vi "Rational Resampling.vi"() -> ()   [LabVIEW 2020]
doc: "This example demonstrates how to use the Rational Resample VI to process a large data sequence consisting of smaller blocks."
uses:
  <vilib>/Utility/error.llb/DialogType.ctl
  <vilib>/Analysis/2dsp.llb/Rational Resample (single channel, DBL).vi
  <vilib>/Analysis/NI_AALPro.lvlib
  <vilib>/Analysis/NI_AALBase.lvlib
panel:
  out "error message":string
  out "Rational Resampling":cluster{"t0":dbl, dbl, "Y":dbl[]}[](graph)
  in  "Stop":bool
  in  "FIR filter specifications":T1={"alias rejection (dB)"=60.0, "normalized bandwidth"=0.42} {"normalized bandwidth" format="%#.6g"; "alias rejection (dB)" format="%#.6g"}
  in  "start index":i32
  in  "resample factor":cluster{"interpolation":i32, "decimation":i32}={"interpolation"=2, "decimation"=7}
  # "Overview This example demonstrates how to use the Rational Resample VI to process a large data sequence consisting of smaller blocks.\nRequirements: LabVIEW Full Development System\nInstructions:\n1. Run the VI.\n2. Change the resample factor parameters and observe the results in the Rational Resampling graph.\n3. Click Stop to stop the VI."
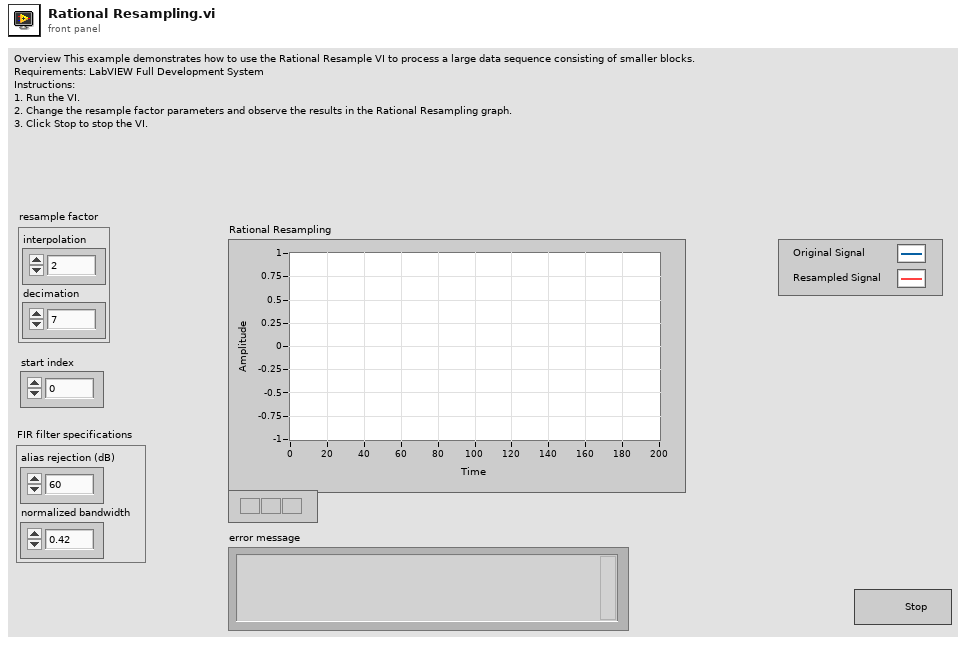
[diagram p1: front panel]
types:
  T1 = cluster{"alias rejection (dB)":dbl, "normalized bandwidth":dbl}
  T2 = typedef "DialogType.ctl" = u16
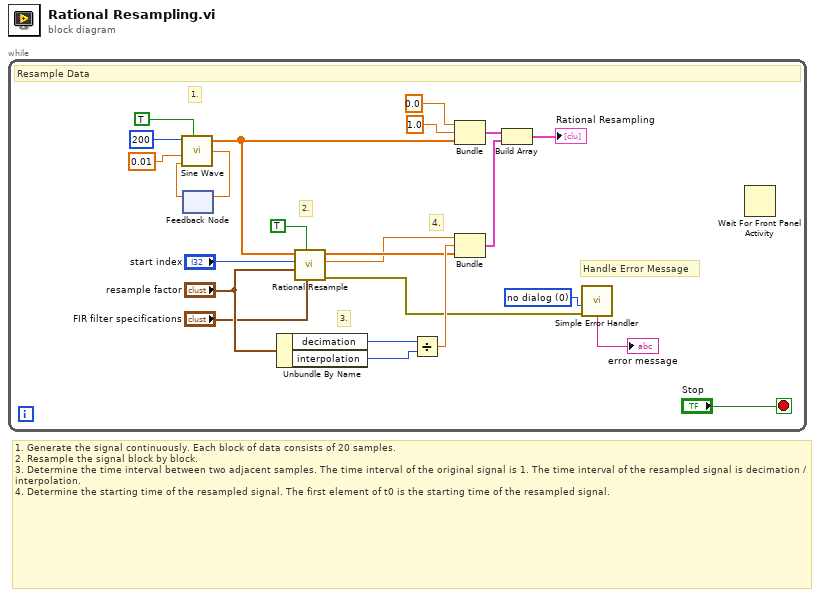
[diagram p0: block diagram]
diagram:
  # "1. Generate the signal continuously. Each block of data consists of 20 samples.\n2. Resample the signal block by block. \n3. Determine the time interval between two adjacent samples. The time interval of the original signal is 1. The time interval of the resampled signal is decimation / interpolation.\n4. Determine the starting time of the resampled signal. The first element of t0 is the starting time of the resampled signal."
  n1 = while {
    stop <- "Stop" stop-if-true
    w6 = T2 0 items=["no dialog", "OK message", "continue or stop message", "OK message + warnings", "continue/stop + warnings"] ("type of dialog (OK msg:1)")
    # "Handle Error Message"
    # "2."
    # "1."
    # "4."
    # "3."
    # "Resample Data"
    n2 = feedback #1() -> (w10:dbl)  [unwired: 1 in]
    n3 = call <vilib>:"Sine Wave.vi"("samples"=200, "frequency"=0.01, "phase in"=w10, "reset phase"=TRUE) -> ("sine wave"=w16:dbl[], "phase out"=w11:dbl)  [unwired: 1 in, 1 out]
    n4 = feedback-in #1(w11) -> ()
    n5 = Unbundle By Name("resample factor") -> ("decimation"=w21:i32, "interpolation"=w1:i32)
    n6 = call-poly <vilib>:"Rational Resample.vi"("FIR filter specifications"="FIR filter specifications", "reset"=TRUE, "resample factor"="resample factor", "start index"="start index", "X"=w16) -> ("error out"=w5:errorcluster, "t0"=w7:dbl, "Y"=w15:dbl[])  [unwired: 4 in]
    n7 = Divide(x=w21, y=w1) -> (x/y=w20:dbl)
    n8 = Bundle(0.0, 1.0, "sine wave"=w16) -> (w24:cluster{dbl, dbl, "sine wave":dbl[]})  [unwired: 1 in]
    n9 = Bundle("t0"=w7, w20, "Y"=w15) -> (w23:cluster{"t0":dbl, dbl, "Y":dbl[]})  [unwired: 1 in]
    n10 = Build Array(w24, w23) -> (→"Rational Resampling":cluster{"t0":dbl, dbl, "Y":dbl[]}[])
    n11 = call <vilib>:"Simple Error Handler.vi"("type of dialog (OK msg:1)"=w6, "error in (no error)"=w5) -> ("message"=→"error message":string)  [unwired: 3 in, 4 out]
    n12 = Wait For Front Panel Activity() -> ()  [unwired: 3 in, 1 out]
  }
